vi "WPI_IMU_ADIS16460_WriteRegister.vi"(8 "error in (no error)":errorcluster, 9 "Data":u16=2049, 10 "ADIS16460 Register":T1=62 items=["PROD_ID"=86, "GLOB_CMD"=62, "DEC_RATE"=54, "FLTR_CTRL"=56, "MSC_CTRL"=50], 11 "SPIDevRef in":T2) -> (0 "error out":errorcluster, 1 "Write OK?":bool, 2 "Register Value":u16, 3 "SPIDevRef out":T2)   [LabVIEW 2015, in "FRC ADIS16460.lvlib"]
uses:
  FRC ADIS16460.lvlib
  <vilib>/Rock Robotics/WPI/SPI/WPI_SPIDevRef.ctl
  <vilib>/Rock Robotics/SystemInterfaces/spilib/spi_bus.ctl
  WPI_IMU_ADIS16460_Registers.ctl
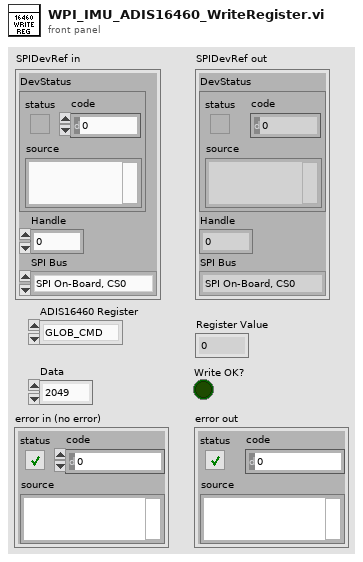
[diagram p1: front panel]
types:
  T1 = typedef "FRC ADIS16460.lvlib/WPI_IMU_ADIS16460_Registers.ctl" = u8
  T2 = typedef "WPI_SPIDevRef.ctl" = cluster{"DevStatus":errorcluster, "Handle":i32, "SPI Bus":T3}
  T3 = typedef "spi_bus.ctl" = enum16{"SPI On-Board, CS0", "SPI On-Board, CS1", "SPI On-Board, CS2", "SPI On-Board, CS3", "SPI MXP", "Invalid"}
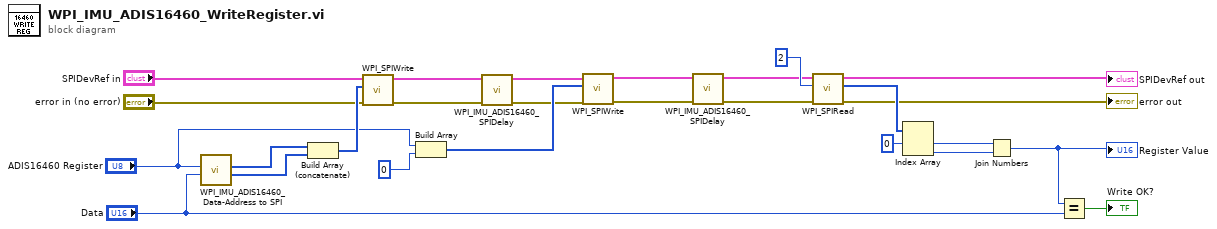
[diagram p0: block diagram]
diagram:
  n1 = call "WPI_IMU_ADIS16460_Data-Address to SPI.vi"("Data"="Data", "Address"="ADIS16460 Register") -> ("Low Word"=w19:u8[], "High Word"=w20:u8[])  [unwired: 8 in]
  n2 = Build Array (concatenate)(w20, w19) -> (w21:u8[])
  n3 = call <vilib>:"WPI_SPIWrite.vi"("error in (no error)"="error in (no error)", "Data To Send"=w21, "SPIDevRef"="SPIDevRef in") -> ("error out"=w7:errorcluster, "SPIDevRef"=w8:T2)  [unwired: 7 out]
  n4 = Build Array("ADIS16460 Register", 0) -> (w18:i32[])
  n5 = call "WPI_IMU_ADIS16460_SPIDelay.vi"("error in"=w7, "SPIDevRef in"=w8) -> ("error out"=w5:errorcluster, "SPIDevRef out"=w6:T2)  [unwired: 8 in]
  n6 = call <vilib>:"WPI_SPIWrite.vi"("error in (no error)"=w5, "Data To Send"=w18, "SPIDevRef"=w6) -> ("error out"=w4:errorcluster, "SPIDevRef"=w3:T2)  [unwired: 7 out]
  n7 = call "WPI_IMU_ADIS16460_SPIDelay.vi"("error in"=w4, "SPIDevRef in"=w3) -> ("error out"=w1:errorcluster, "SPIDevRef out"=w2:T2)  [unwired: 8 in]
  n8 = call <vilib>:"WPI_SPIRead.vi"("error in (no error)"=w1, "Num to Read"=2, "SPIDevRef"=w2) -> ("error out"=→"error out":errorcluster, "Received Data"=w24:u8[], "SPIDevRef"=→"SPIDevRef out":T2)  [unwired: 6 in]
  n9 = Index Array(array=w24, index #1=0 ("index")) -> (element #1=w16:u8, element #2=w15:u8)  [unwired: 1 in]
  n10 = Join Numbers(hi=w16, lo=w15) -> ((hi.lo)=w14:u16)
  "Register Value" <- w14
  n11 = Equal?(x=w14, y="Data") -> (x = y?=→"Write OK?":bool)
